vi "DPR250DriverServer.vi"   [LabVIEW 2010, in "DPR250.lvlib"]
uses:
  DPR250.lvlib
  Comunication Status.ctl
  <vilib>/Instr/_visa.llb/VISA Configure Serial Port (Instr).vi
types:
  T1 = enum32{"Invalid", "Standard", "Closed", "Hidden", "Minimized", "Maximized"}
  T2 = typedef "DPR250.lvlib/Comunication Status.ctl" = string
  T3 = typedef "DPR250.lvlib/Serial Config.ctl" = cluster{"串口选择":refnum<visa-resource-name>, "通讯速率":u32, "超时时间":u32, "数据位长":u16, "奇偶校验":enum16{"None", "Odd", "Even", "Mark", "Space"}, "停止位长":u16, "握手控制":u16, "字符结束":bool, "结束字符":u8, "仪器地址":u8}
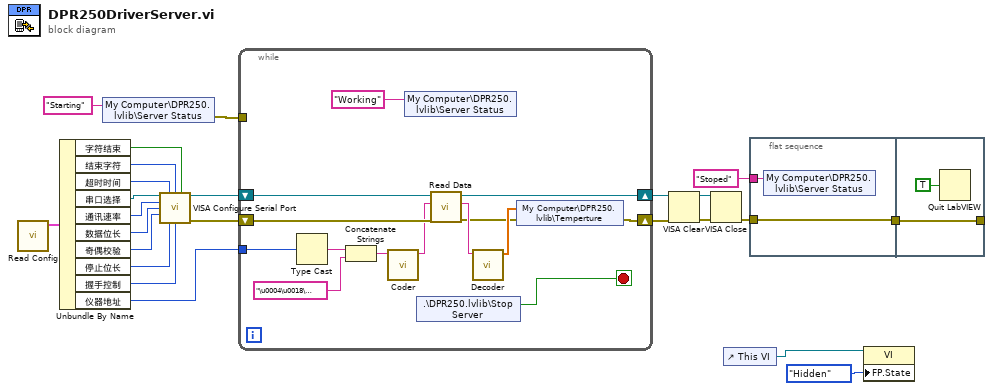
[diagram p0: block diagram]
diagram:
  n1 = call "Read Config.vi"() -> ("value"=w22:T3)  [unwired: 10 in, 1 out]
  n2 = Unbundle By Name(w22) -> ("字符结束"=w11:bool, "结束字符"=w10:u8, "超时时间"=w9:u32, "串口选择"=w21:refnum<visa-resource-name>, "通讯速率"=w20:u32, "数据位长"=w19:u16, "奇偶校验"=w18:enum16{"None", "Odd", "Even", "Mark", "Space"}, "停止位长"=w17:u16, "握手控制"=w16:u16, "仪器地址"=w14:u8)
  n3 = shared-variable "My Computer\\DPR250.lvlib\\Server Status"(T2 "Starting" ("Server Status")) -> (error out=w4:errorcluster)  [unwired: 1 in]
  n4 = call-poly "VISA Configure Serial Port"("VISA resource name"=w21, "timeout (10sec)"=w9, "termination char\n(0xA = '\\n' = LF)"=w10, "Enable Termination\nChar (T)"=w11, "baud rate (9600)"=w20, "data bits (8)"=w19, "parity (0:none)"=w18, "stop bits (10: 1 bit)"=w17, "flow control (0:none)"=w16) -> ("VISA resource name out"=w15:refnum<visa-resource-name>, "error out"=w5:errorcluster)  [unwired: 1 in, 4 out]
  n5 = while {
    shift-right: [w37] -> w13
    shift-left: w15 -> [w36]
    tunnel: w14 -> [w35]
    shift-right: [w30] -> w7
    shift-left: w5 -> [w29]
    tunnel: w4 -> [_]
    stop <- w25 stop-if-true
    n6 = Type Cast(x=w35) -> (*(type *) &x=w34:string)  [unwired: 1 in]
    n7 = Concatenate Strings(w34, "\u0004\u0018\u0000\u0000(" ("Input")) -> (w26:string)
    n8 = call "Coder.vi"("Input"=w26) -> ("Output"=w27:string)  [unwired: 10 in]
    n9 = shared-variable "My Computer\\DPR250.lvlib\\Server Status"(T2 "Working" ("Server Status")) -> ()  [unwired: 1 in, 1 out]
    n10 = shared-variable ".\\DPR250.lvlib\\Stop Server"() -> (w25:bool)  [unwired: 1 in, 1 out]
    n11 = call "Read Data.vi"("error in (no error)"=w29, "COMMAND"=w27, "VISA resource name in"=w36) -> ("error out"=w28:errorcluster, "Output"=w32:string, "VISA resource name out"=w37:refnum<visa-resource-name>)  [unwired: 6 in]
    n12 = call "Decoder.vi"("Input"=w32) -> ("Data"=w31:sgl[])  [unwired: 10 in]
    n13 = shared-variable "My Computer\\DPR250.lvlib\\Temperture"(w31, error in=w28) -> (error out=w30:errorcluster)
  }
  n14 = VISA Clear(VISA resource name=w13, error in (no error)=w7) -> (VISA resource name out=w12:refnum<visa-resource-name>, error out=w6:errorcluster)
  n15 = VISA Close(VISA resource name=w12, error in (no error)=w6) -> (error out=w8:errorcluster)
  n16 = control-ref of="This VI"() -> (w2:refnum<vi>)
  n17 = flat-sequence {
    tunnel: T2 "Stoped" ("Server Status") -> [w40]
    tunnel: w8 -> [w39]
    tunnel: [w39] -> w3
    tunnel: [w42] -> _
    tunnel: w3 -> [w42]
    frame #0 {
      n18 = shared-variable "My Computer\\DPR250.lvlib\\Server Status"(w40) -> ()  [unwired: 1 in, 1 out]
    }
    frame #1 {
      n19 = Quit LabVIEW(quit? (T)=TRUE) -> ()
    }
  }
  n20 = property class="VI"(reference=w2, "FP.State"=T1."Hidden" ("Front Panel Window:State")) -> ()  [unwired: 1 in, 2 out]
